vi "DatabaseRead SubVI.vi"(8 "error in (no error)":errorcluster, 11 "File name":string) -> (0 "error out":errorcluster, 3 "UserName":string)   [LabVIEW 2024]
doc: "SubVi odpowiedzialne za odczytywanie wartości z bazy danych.\n\nKonieczne jest samodzielne podłączenie wygenerowanego Microsoft DataLink"
uses:
  <vilib>/Utility/error.llb/Trim Whitespace One-Sided.vi
  <vilib>/addons/database/_DB Variant To Data/Database Variant To Data.xnode
  <vilib>/addons/database/Connection.llb/DB Tools Open Connec (Path).vi
  <vilib>/addons/database/NI_Database_API.lvlib
panel:
  out "subarray":string[](array[string])
  in  "connection information":path
  out "data":string[][](array[string])
  # "Wzorzec"
  # "Porownanie"
  # "Wynik"
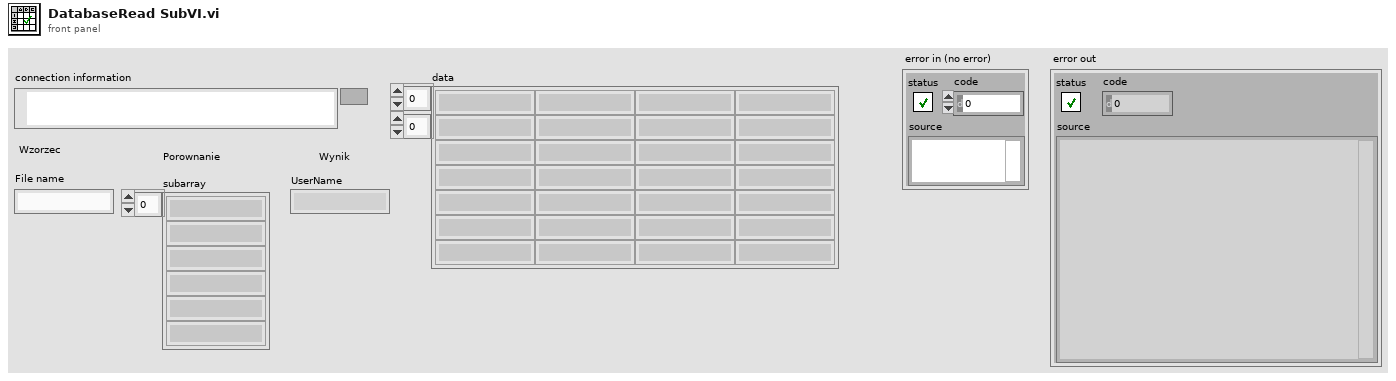
[diagram p1: front panel]
types:
  T1 = typedef "NI_Database_API.lvlib/Conn ObjectReference.ctl" = refnum<k1>
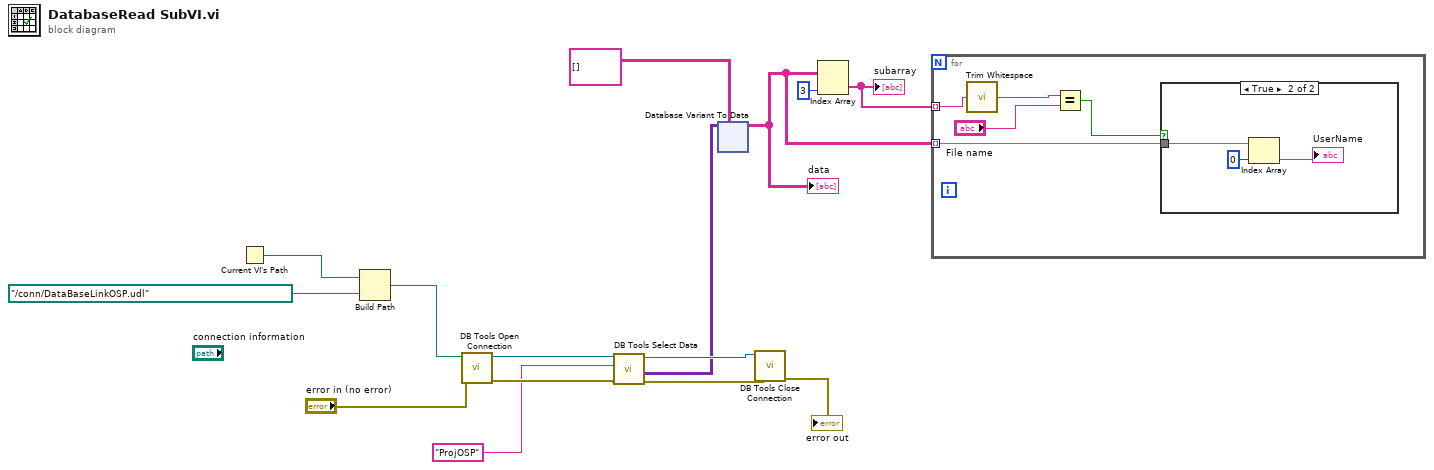
[diagram p0: block diagram]
diagram:
  n1 = Current VI's Path() -> (path=w3:path)
  n2 = Build Path(base path=w3, name or relative path=path "../conn/DataBaseLinkOSP.udl") -> (appended path=w1:path)
  n3 = call-poly <vilib>:"DB Tools Open Connection.vi"("error in (no error)"="error in (no error)", "connection information"=w1) -> ("error out"=w13:errorcluster, "connection reference"=w15:T1)  [unwired: 6 in]
  n4 = call <vilib>:"DB Tools Select Data.vi"("error in (no error)"=w13, "table"="ProjOSP", "connection reference"=w15) -> ("error out"=w12:errorcluster, "data"=w10:variant[][], "connection reference out"=w14:T1)  [unwired: 3 in]
  n5 = xnode "Database Variant To Data"("database variant"=w10, "type"=string[][] []) -> ("data"=w4:string[][])  [unwired: 1 in, 1 out]
  "data" <- w4
  n6 = call <vilib>:"DB Tools Close Connection.vi"("error in (no error)"=w12, "connection reference"=w14) -> ("error out"=→"error out":errorcluster)  [unwired: 5 in]
  n7 = Index Array(array=w4, index (col)=3 ("disabled index (col)")) -> (element=w5:string[])  [unwired: 1 in]
  "subarray" <- w5
  n8 = for {
    tunnel: w5 -> [w17] mode=indexing
    tunnel: w4 -> [w16] mode=indexing
    n9 = call <vilib>:"Trim Whitespace.vi"("string"=w17) -> ("trimmed string"=w20:string)  [unwired: 1 in]
    n10 = Equal?(x=w20, y="File name") -> (x = y?=w18:bool)
    n11 = case shown="True" w18 {
      tunnel: w16 -> [_ w23]
      frame False {
      }
      frame True {
        n12 = Index Array(array=w23, index=0) -> (element=→"UserName":string)
      }
    }
  }
